vi "Pixie4Boot.vi"(1 "Select PXI chassis type":string(combo)="4 or 8-slot chassis", 2 "Offline analysis ?":bool, 3 "Module #":i16[](array[numeric])=[3, 4] caption="PXI Slot #" min=2 max=18 step=1, 4 "Total number of Pixie-4 modules":i16=1 min=1 max=17 step=1, 5 "DSP memory variable file (.lst file in folder \"DSP\")":path=path "C:/Program Files/National Instruments/LabVIEW 2009/user.lib/DSP/PXIcode.lst", 6 "DSP I/O variable file (.var file in folder \"DSP\")":path=path "C:/Program Files/National Instruments/LabVIEW 2009/user.lib/DSP/PXIcode.var", 7 "DSP parameters file (.set file in folder \"Configuration\")":path=path "C:/Documents and Settings/Administrator/Desktop/dsp files/36Cl/oct 2013/1st.set", 8 "DSP executable code file (.bin file in folder DSP\")":path=path "C:/Program Files/National Instruments/LabVIEW 2009/user.lib/DSP/PXIcode.bin", 9 "Signal proceesing FPGA file (.bin file in folder \"Firmware\")":path=path "C:/Program Files/National Instruments/LabVIEW 2009/user.lib/Firmware/pixie.bin", 10 "Communication FPGA file for REVC (.bin file in folder \"Firmware\")":path=path "C:/Program Files/National Instruments/LabVIEW 2009/user.lib/Firmware/syspixie_revC.bin", 11 "Communication FPGA file for REVB (.bin file in folder \"Firmware\")":path=path "C:/Program Files/National Instruments/LabVIEW 2009/user.lib/Firmware/syspixie_RevB.bin") -> (0 "Return value for booting":i32)   [LabVIEW 2016]
uses:
  Drivers/Pixie4DLL.dll
panel:
  in  "Boolean":bool
  in  "stop":bool
  # "0  - boot successful\n-1  - unable to scan the PXI crate slots\n-2  - unable to read communication FPGA configuration (Rev. B)\n-3  - unable to read communication FPGA configuration (Rev. C)\n-4  - unable to read signal processing FPGA configuration\n-5  - unable to read DSP executable code\n-6  - unable to read DSP parameter values\n-7  - unable to initialize DSP parameter names\n-8  - failed to boot all modules present in the system\n-9  - failed to initialize NUMBER_MODULES\n-10- failed to initialize OFFLINE_ANALYSIS\n-11- failed to initialize MAX_NUMBER_MODULES\n-12- failed to initialize SLOT_WAVE"
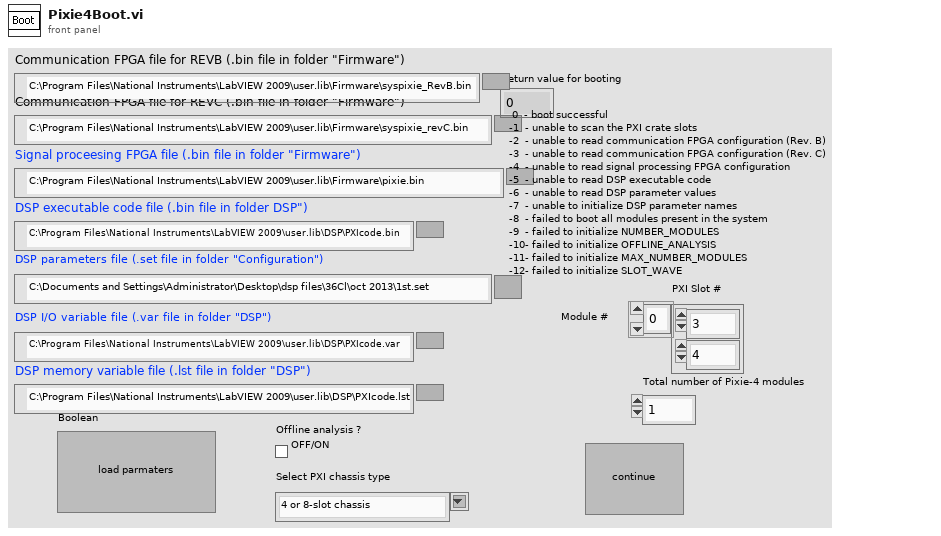
[diagram p1: front panel]
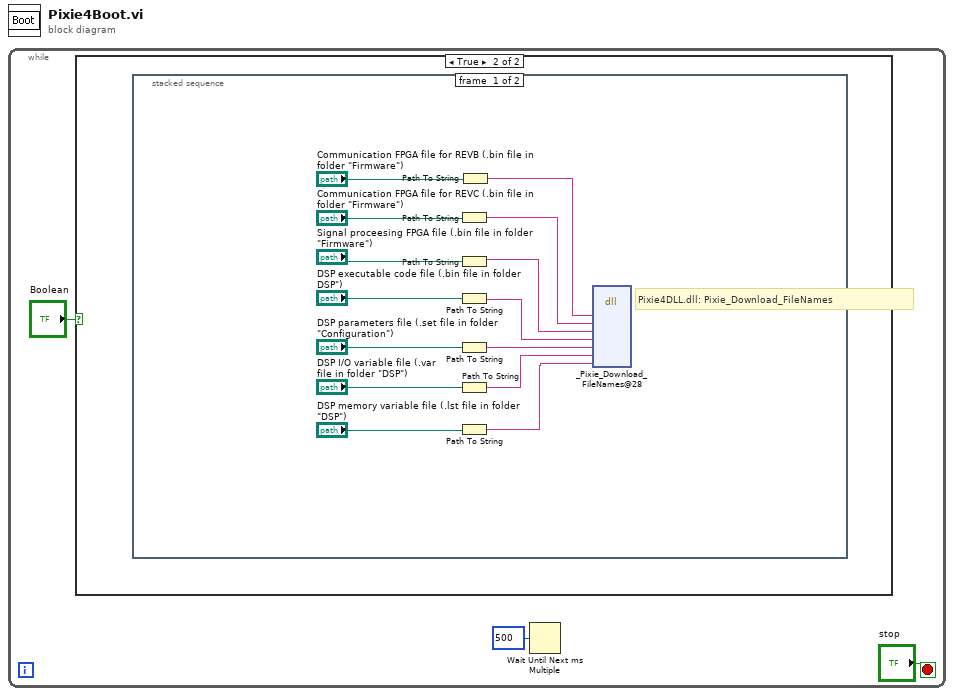
[diagram p0: block diagram]
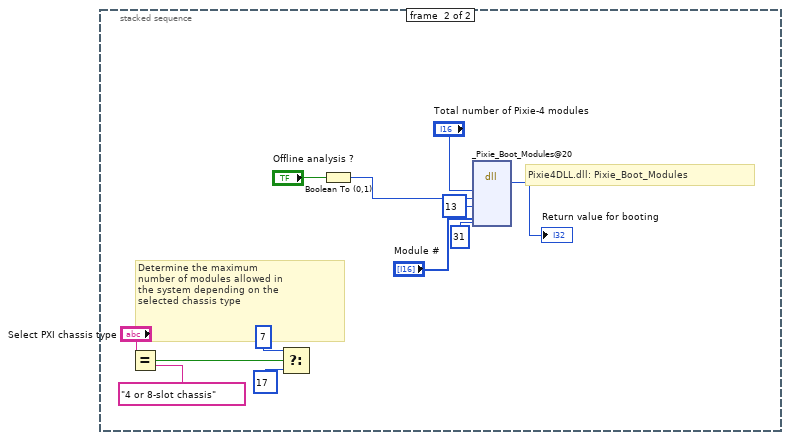
[diagram p3: hidden frame]
diagram:
  n1 = while {
    stop <- "stop" stop-if-true
    n2 = case shown="True" "Boolean" {
      frame False {
      }
      frame True {
        n3 = stacked-sequence {
          frame #0 {
            # "Pixie4DLL.dll: Pixie_Download_FileNames"
            n4 = Path To String(path="Communication FPGA file for REVC (.bin file in folder \"Firmware\")") -> (string=w6:string)
            n5 = Path To String(path="Signal proceesing FPGA file (.bin file in folder \"Firmware\")") -> (string=w7:string)
            n6 = Path To String(path="DSP executable code file (.bin file in folder DSP\")") -> (string=w8:string)
            n7 = Path To String(path="DSP parameters file (.set file in folder \"Configuration\")") -> (string=w9:string)
            n8 = Path To String(path="DSP I/O variable file (.var file in folder \"DSP\")") -> (string=w10:string)
            n9 = Path To String(path="DSP memory variable file (.lst file in folder \"DSP\")") -> (string=w11:string)
            n10 = Path To String(path="Communication FPGA file for REVB (.bin file in folder \"Firmware\")") -> (string=w4:string)
            n11 = dll-call lib="D:/Users/wymanm/Desktop/DAQuiri - 2017a/lois/Drivers/Pixie4DLL.dll" fn="_Pixie_Download_FileNames@28" label="Call Library Function"("ComFPGAFileNameRevB"=w4, "ComFPGAFileNameRevC"=w6, "SPFPGAFileName"=w7, "DSPCodeFileName"=w8, "DSPParFileName"=w9, "DSPVarFileName"=w10, "DSPLstFileName"=w11) -> ()  [unwired: 11 in, 2 out]
          }
          frame #1 {
            # "Pixie4DLL.dll: Pixie_Boot_Modules"
            # "Determine the maximum\nnumber of modules allowed in\nthe system depending on the\nselected chassis type"
            n12 = Equal?(x="Select PXI chassis type", y="4 or 8-slot chassis") -> (x = y?=w20:bool)
            n13 = Select(t=7, s=w20, f=17) -> ()  [unwired: 1 out]
            n14 = Boolean To (0,1)(Boolean="Offline analysis ?") -> (0, 1=w26:i16)
            n15 = dll-call lib="D:/Users/wymanm/Desktop/DAQuiri - 2017a/lois/Drivers/Pixie4DLL.dll" fn="_Pixie_Boot_Modules@20" label="Call Library Function"("TotalNumberModules"="Total number of Pixie-4 modules", "OfflineAnalysis"=w26, "MaxNumberOfModules"=u16 13, "PXISlotMap"="Module #", "BootPattern"=31) -> ("return type"=→"Return value for booting":i32)  [unwired: 8 in, 2 out]
          }
        }
      }
    }
    n16 = Wait Until Next ms Multiple(millisecond multiple=u32 500) -> ()  [unwired: 1 out]
  }
